vi "PhotonVision_Aim_And_Range.vi"(8 "Init":bool, 9 "AprilTagID":i32, 10 "Use AprilTag":bool, 11 "CameraName":string) -> (1 "Right Motor Value":dbl, 3 "Left Motor Value":dbl)   [LabVIEW 2019]
uses:
  <vilib>/Rock Robotics/WPI/ThirdParty/PhotonVisionLib/PhotonVisionLib.lvlib
  C:/Program Files/National Instruments/LabVIEW 2019/Targets/NI/RT/vi.lib/Rock Robotics/WPI/Joystick/WPI_JoystickArcadeMapping.vi
  <vilib>/Rock Robotics/WPI/ThirdParty/JAS_Junk/TrajLib/Trajectory_Library.lvlib
  <vilib>/Rock Robotics/Network Tables/NT Write Number.vi
  <vilib>/Rock Robotics/Network Tables/NT Write Boolean.vi
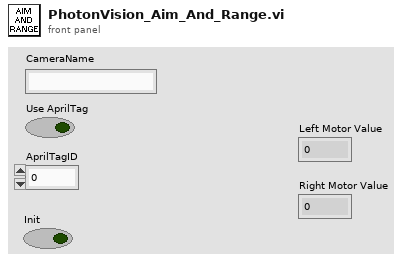
[diagram p1: front panel]
types:
  T1 = typedef "PhotonVisionLib.lvlib/PhotonPipelineResultType.ctl" = cluster{"Targets":T2[], "PhotonMultiTargetPNPResult":T8, "PhotonPipelineMetadata":T10}
  T2 = typedef "PhotonVisionLib.lvlib/PhotonTrackedTargetType.ctl" = cluster{"Yaw":dbl, "Pitch":dbl, "Area":dbl, "Skew":dbl, "MinAreaRectCorners":T3[], "BestCameraToTarget":T4, "FiducialId":i32, "AltCameraToTarget":T4, "PoseAmbiguity":dbl, "DetectedCorners":T3[], "ObjDetectId":i32, "ObjDetectConf":sgl}
  T3 = typedef "PhotonVisionLib.lvlib/TargetCornerType.ctl" = cluster{"X":dbl, "Y":dbl}
  T4 = typedef "Trajectory_Library.lvlib/TRANSFORM3D.ctl" = cluster{"TRANSLATION3D":T5, "ROTATION3D":T6, "XF":bool}
  T5 = typedef "Trajectory_Library.lvlib/TRANSLATION3D.ctl" = cluster{"X":dbl, "Y":dbl, "Z":dbl}
  T6 = typedef "Trajectory_Library.lvlib/ROTATION3D.ctl" = cluster{"Q_quaternion":T7}
  T7 = typedef "Trajectory_Library.lvlib/QUATERNION.ctl" = cluster{"R":dbl, "V":dbl[]}
  T8 = typedef "PhotonVisionLib.lvlib/PhotonMultiTargetPNPResultType.ctl" = cluster{"PhotonPNPResult":T9, "FiducialIDsUsed":i16[]}
  T9 = typedef "PhotonVisionLib.lvlib/PhotonPNPResultType.ctl" = cluster{"IsPresent":bool, "bestReprojErr":dbl, "altReprojErr":dbl, "ambiguity":dbl, "Best":T4, "Alt":T4}
  T10 = typedef "PhotonVisionLib.lvlib/PhotonPipelineMetadataType.ctl" = cluster{"CaptureTimestampMicros":i64, "PublishTimestampMicros":i64, "SequenceID":i64, "TimeSinceLastPong":i64}
  T11 = typedef "Trajectory_Library.lvlib/PID_ADV_LIMITS.ctl" = cluster{"MaxInput":dbl, "MinInput":dbl, "Continuous":bool, "MaxOutput":dbl, "MinOutput":dbl}
  T12 = typedef "Trajectory_Library.lvlib/PID_ADV_TUNING.ctl" = cluster{"Kf":dbl, "Kp":dbl, "Ki":dbl, "Kd":dbl, "MaximumIntegral":dbl, "MinimumIntegral":dbl, "Filter Derivative":bool, "IntegralZone":dbl}
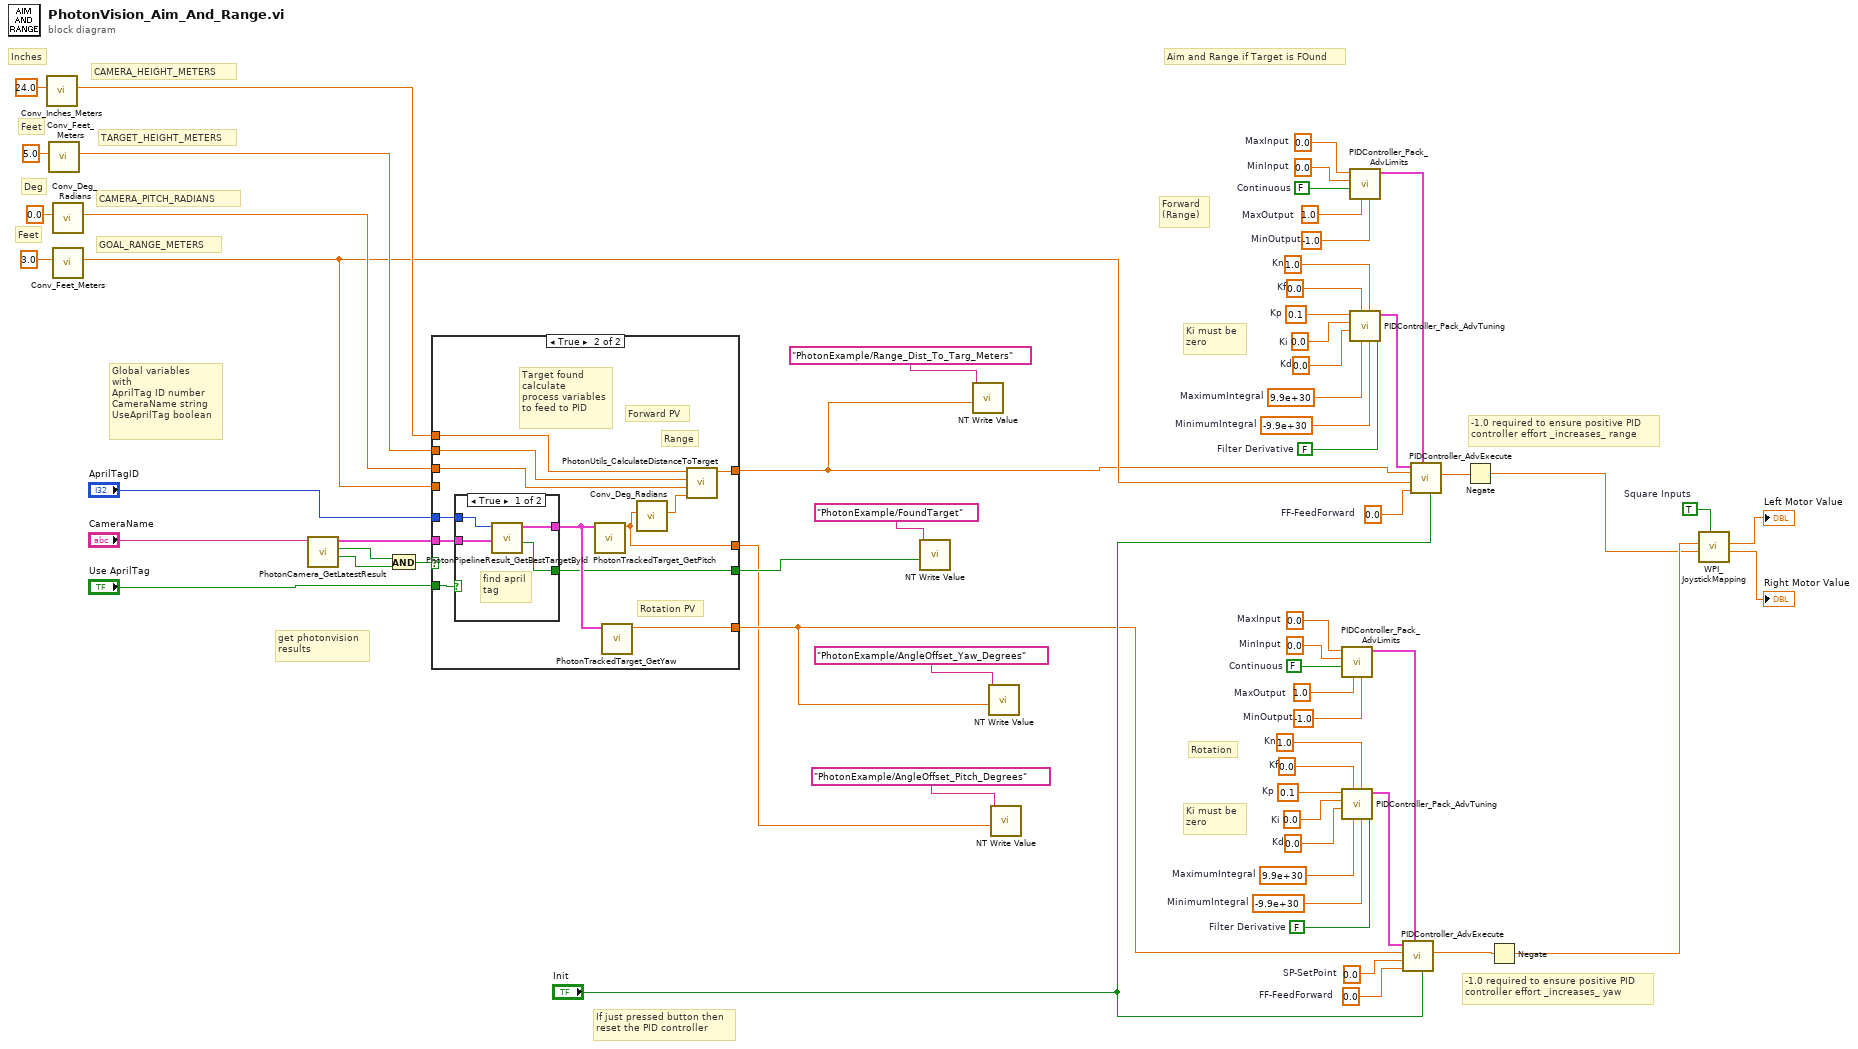
[diagram p0: block diagram]
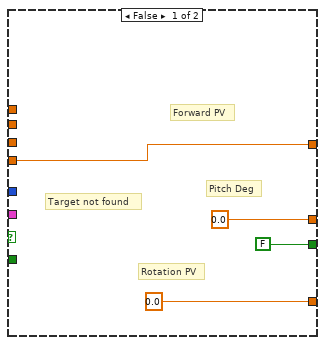
[diagram p2: hidden frame]
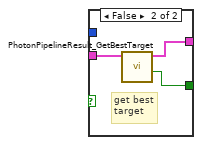
[diagram p3: hidden frame]
diagram:
  w50 = 0.0  # FF-FeedForward
  w49 = 0.0  # FF-FeedForward
  w47 = 0.0  # SP-SetPoint
  w31 = 1.0  # Kn
  w32 = 0.1  # Kp
  w33 = 0.0  # Ki
  w34 = 0.0  # Kd
  w35 = 0.0  # Kf
  w36 = 9.9e+30  # MaximumIntegral
  w37 = -9.9e+30  # MinimumIntegral
  w38 = FALSE  # Filter Derivative
  w40 = 0.0  # MinInput
  w41 = FALSE  # Continuous
  w42 = 1.0  # MaxOutput
  w39 = -1.0  # MinOutput
  w43 = 0.0  # MaxInput
  w16 = 1.0  # Kn
  w17 = 0.1  # Kp
  w18 = 0.0  # Ki
  w19 = 0.0  # Kd
  w20 = 0.0  # Kf
  w21 = 9.9e+30  # MaximumIntegral
  w22 = -9.9e+30  # MinimumIntegral
  w23 = FALSE  # Filter Derivative
  w25 = 0.0  # MinInput
  w26 = FALSE  # Continuous
  w27 = 1.0  # MaxOutput
  w24 = -1.0  # MinOutput
  w28 = 0.0  # MaxInput
  w13 = TRUE  # Square Inputs
  # "Global variables\nwith \nAprilTag ID number\nCameraName string\nUseAprilTag boolean"
  # "Feet"
  # "Deg"
  # "Feet"
  # "Inches"
  # "GOAL_RANGE_METERS"
  # "CAMERA_PITCH_RADIANS"
  # "TARGET_HEIGHT_METERS"
  # "CAMERA_HEIGHT_METERS"
  # "Aim and Range if Target is FOund"
  # "-1.0 required to ensure positive PID \ncontroller effort _increases_ range"
  # "-1.0 required to ensure positive PID \ncontroller effort _increases_ yaw"
  # "Ki must be \nzero"
  # "Ki must be \nzero"
  # "If just pressed button then\nreset the PID controller"
  # "Rotation"
  # "Forward \n(Range)"
  # "get photonvision\nresults"
  n1 = call <vilib>:"Conv_Inches_Meters.vi"("INCH"=24.0) -> ("Meters"=w64:dbl)  [unwired: 10 in]
  n2 = call <vilib>:"Conv_Feet_Meters.vi"("Feet"=5.0) -> ("Meters"=w63:dbl)  [unwired: 10 in]
  n3 = call <vilib>:"Conv_Deg_Radians.vi"("Degress"=0.0) -> ("Radians"=w62:dbl)  [unwired: 10 in]
  n4 = call <vilib>:"Conv_Feet_Meters.vi"("Feet"=3.0) -> ("Meters"=w61:dbl)  [unwired: 10 in]
  n5 = call <vilib>:"PhotonCamera_GetLatestResult.vi"("CameraName"="CameraName") -> ("New Data"=w3:bool, "HasTargets"=w4:bool, "PipelineResult"=w46:T1)  [unwired: 6 in, 2 out]
  n6 = And(x=w4, y=w3) -> (x .and. y?=w5:bool)
  n7 = case shown="True" w5 {
    tunnel: w46 -> [_ w80]
    tunnel: [w67 w77] -> w6
    tunnel: [0.0 w76] -> w8
    tunnel: w64 -> [_ w73]
    tunnel: w63 -> [_ w74]
    tunnel: w62 -> [_ w75]
    tunnel: w61 -> [w67 _]
    tunnel: "Use AprilTag" -> [_ w72]
    tunnel: [FALSE ("TargetFound") w71] -> w56
    tunnel: "AprilTagID" -> [_ w70]
    tunnel: [0.0 ("Pitch") w69] -> w1
    frame False {
      # "Pitch Deg"
      # "Forward PV"
      # "Rotation PV"
      # "Target not found"
    }
    frame True {
      # "Target found\ncalculate\nprocess variables\nto feed to PID"
      # "Range"
      # "Forward PV"
      # "Rotation PV"
      n8 = case shown="True" w72 {
        tunnel: w80 -> [w82 w87]
        tunnel: [w84 w86] -> w78
        tunnel: [w83 w85] -> w71
        tunnel: w70 -> [w81 _]
        frame True {
          # "find april\ntag"
          n9 = call <vilib>:"PhotonPipelineResult_GetBestTargetById.vi"("PhotonPipelineResult"=w82, "FiducialId"=w81) -> ("Target Found"=w83:bool, "PhotonTrackedTarget"=w84:T2)  [unwired: 7 in, 1 out]
        }
        frame False {
          # "get best\ntarget"
          n10 = call <vilib>:"PhotonPipelineResult_GetBestTarget.vi"("PhotonPipelineResult"=w87) -> ("TargetFound"=w85:bool, "PhotonTrackedTarget"=w86:T2)  [unwired: 9 in]
        }
      }
      n11 = call <vilib>:"PhotonTrackedTarget_GetPitch.vi"("TrackedTarget"=w78) -> ("Pitch"=w69:dbl)  [unwired: 10 in]
      n12 = call <vilib>:"PhotonTrackedTarget_GetYaw.vi"("TrackedTarget"=w78) -> ("Yaw"=w76:dbl)  [unwired: 10 in]
      n13 = call <vilib>:"Conv_Deg_Radians.vi"("Degress"=w69) -> ("Radians"=w79:dbl)  [unwired: 10 in]
      n14 = call <vilib>:"PhotonUtils_CalculateDistanceToTarget.vi"("TargetPitch_Radians"=w79, "CameraPitch_Radians"=w75, "TargetHeight_Meters"=w74, "CameraHeight_Meters"=w73) -> ("DistanceToTarget_Meters"=w77:dbl)  [unwired: 7 in]
    }
  }
  n15 = call-poly <vilib>:"NT Write Value.vi"("value"=w56, "name"="PhotonExample/FoundTarget" ("Name")) -> ()  [unwired: 9 in, 1 out]
  n16 = call-poly <vilib>:"NT Write Value.vi"("value"=w6, "name"="PhotonExample/Range_Dist_To_Targ_Meters" ("Name")) -> ()  [unwired: 9 in, 1 out]
  n17 = call-poly <vilib>:"NT Write Value.vi"("value"=w8, "name"="PhotonExample/AngleOffset_Yaw_Degrees" ("Name")) -> ()  [unwired: 9 in, 1 out]
  n18 = call-poly <vilib>:"NT Write Value.vi"("value"=w1, "name"="PhotonExample/AngleOffset_Pitch_Degrees" ("Name")) -> ()  [unwired: 9 in, 1 out]
  n19 = call <vilib>:"PIDController_Pack_AdvLimits.vi"("MinOutput"=w39, "MaxOutput"=w42, "Continuous"=w41, "MinInput"=w40, "MaxInput"=w43) -> ("Adv PID Limits"=w45:T11)  [unwired: 6 in]
  n20 = call <vilib>:"PIDController_Pack_AdvTuning.vi"("Filter Derivative"=w38, "MinimumIntegral"=w37, "Kn"=w31, "MaximumIntegral"=w36, "Kf"=w35, "Kd"=w34, "Ki"=w33, "Kp"=w32) -> ("Adv PID Tuning"=w44:T12)  [unwired: 3 in]
  n21 = call <vilib>:"PIDController_Pack_AdvLimits.vi"("MinOutput"=w24, "MaxOutput"=w27, "Continuous"=w26, "MinInput"=w25, "MaxInput"=w28) -> ("Adv PID Limits"=w30:T11)  [unwired: 6 in]
  n22 = call <vilib>:"PIDController_Pack_AdvTuning.vi"("Filter Derivative"=w23, "MinimumIntegral"=w22, "Kn"=w16, "MaximumIntegral"=w21, "Kf"=w20, "Kd"=w19, "Ki"=w18, "Kp"=w17) -> ("Adv PID Tuning"=w29:T12)  [unwired: 3 in]
  n23 = call <vilib>:"PIDController_AdvExecute.vi"("Reset"="Init", "Adv PID Limits"=w45, "FF-FeedForward"=w50, "SP-SetPoint"=w47, "PV-Measurement"=w8, "Adv PID Tuning"=w44) -> ("CO-ControlOutput"=w53:dbl)  [unwired: 3 in, 2 out]
  n24 = call <vilib>:"PIDController_AdvExecute.vi"("Reset"="Init", "Adv PID Limits"=w30, "FF-FeedForward"=w49, "SP-SetPoint"=w61, "PV-Measurement"=w6, "Adv PID Tuning"=w29) -> ("CO-ControlOutput"=w51:dbl)  [unwired: 3 in, 2 out]
  n25 = Negate(x=w51) -> (-x=w52:dbl)
  n26 = Negate(x=w53) -> (-x=w54:dbl)
  n27 = call-poly <vilib>:"WPI_JoystickMapping.vi"("Square Inputs"=w13, "Y axis value"=w52, "X axis value"=w54) -> ("Right Motor Value"=→"Right Motor Value":dbl, "Left Motor Value"=→"Left Motor Value":dbl)  [unwired: 7 in]
